vi "SUB_WriteRTC.vi"(2 "DATA_TIME":string, 3 "telnet connection":T1) -> (0 "data out":string, 1 "OK ?":bool)   [LabVIEW 2011]
uses:
  <vilib>/addons/internet/telnet/telnet.llb/Telnet Session.ctl
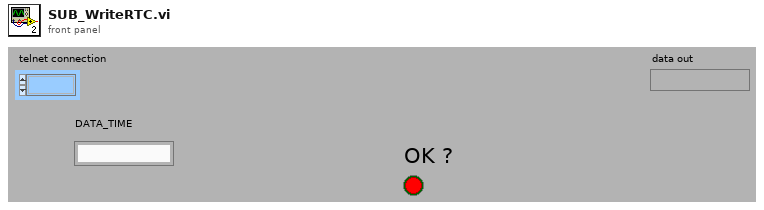
[diagram p1: front panel]
types:
  T1 = typedef "Telnet Session.ctl" = refnum<k1>
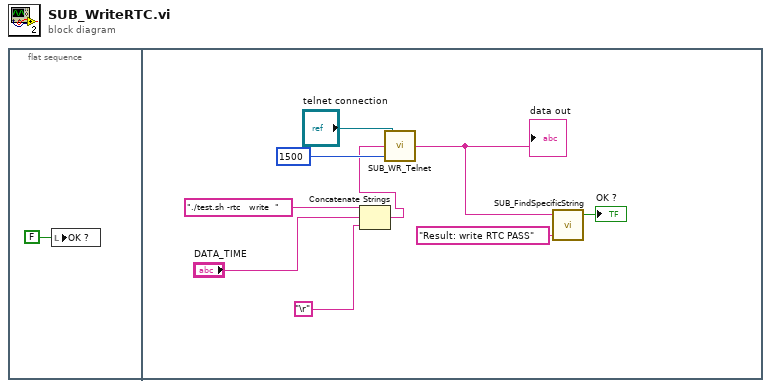
[diagram p0: block diagram]
diagram:
  n1 = flat-sequence {
    frame #0 {
      n2 = local write "OK ?"(FALSE ("OK ?")) -> ()
    }
    frame #1 {
      n3 = Concatenate Strings("./test.sh -rtc   write  ", "DATA_TIME", "\r") -> (w8:string)
      n4 = call "SUB_WR_Telnet.vi"("timeout ms"=1500, "data in"=w8, "telnet connection"="telnet connection") -> ("data out"=w6:string)  [unwired: 1 in, 1 out]
      "data out" <- w6
      n5 = call "SUB_FindSpecificString.vi"("Find this String"="Result: write RTC PASS", "String data"=w6) -> ("Found"=→"OK ?":bool)  [unwired: 2 in, 1 out]
    }
  }
